vi "BundleMagic.vi"(6 "Mouse Position":cluster{"Left":i32, "Top":i32}, 7 "User VI Ref":refnum<vi>, 8 "Is Multi-select?":bool, 9 "Remaining Items":refnum<vi>[](array[refnum]), 10 "Affected Items":T2, 11 "Menu Refnum":refnum<k9>) -> (3 "Menu Items To Add":T1(array[cluster]))   [LabVIEW 2023]
doc: "This VI is part of a plug-in for modifying the LabVIEW shortcut menus. This is the builder VI which is called when the shortcut menu is built. It tells LabVIEW which shortcut menu items to add to the menu."
uses:
  BundleMagic.ctl
panel:
  # "FIX_NEXT_ISSUE BRANCH"
  # "Rules a popup plug-in must follow:\n* This VI's file name must match the file name of the LLB -- only the file extensions should be different.\n* This VI must have debugging disabled or it will be ignored as a plug-in.\n* For all menu items, \"tag suffix + file name of this VI\" must be less than 240 characters.\n* You can disconnect the \"Affected Items\" from the typedef to make the plug-in load faster. The typedef is only there to assist you in keeping this VI and the execution VI using to the same type.\n* All controls on this panel except \"Affected Items\" are locked to prevent accidental edits. Do not change the types or the names of controls other than the elements inside the \"Affected Items\" cluster.\n* See Context Help for more information on the individual controls."
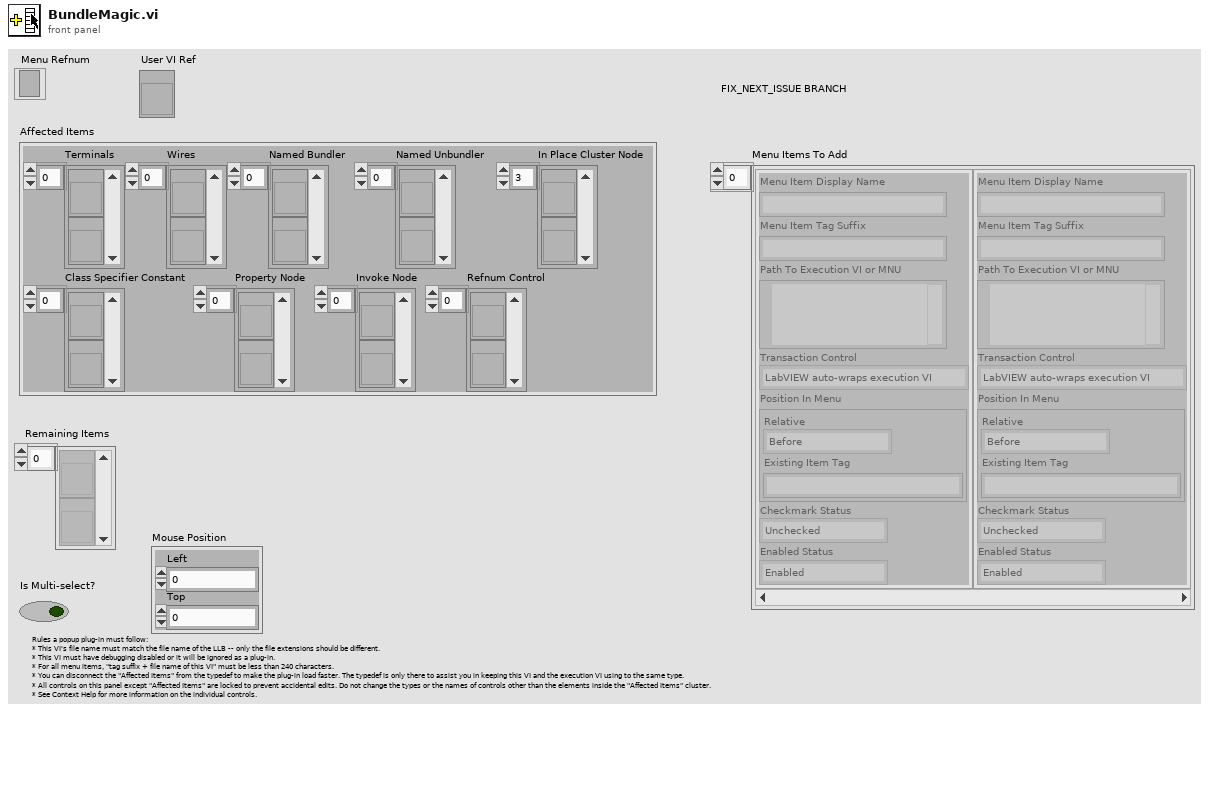
[diagram p1: front panel]
types:
  T1 = cluster{"Menu Item Display Name":string, "Menu Item Tag Suffix":string, "Path To Execution VI or MNU":path, "Transaction Control":enum8{"LabVIEW auto-wraps execution VI", "Execution VI will define if needed"}, "Position In Menu":cluster{"Relative":enum8{"Before", "Instead of", "After", "Into Submenu"}, "Existing Item Tag":string}, "Checkmark Status":enum8{"Unchecked", "Checked"}, "Enabled Status":enum8{"Enabled", "Disabled"}}[]
  T2 = typedef "BundleMagic.ctl" = cluster{"Terminals":refnum<vi>[], "Wires":refnum<vi>[], "Named Bundler":refnum<vi>[], "Named Unbundler":refnum<vi>[], "In Place Cluster Node":refnum<vi>[], "Class Specifier Constant":refnum<vi>[], "Property Node":refnum<vi>[], "Invoke Node":refnum<vi>[], "Refnum Control":refnum<vi>[]}
  T3 = enum16{"[NONE]", "Cluster Wire", "Named Un/Bundler", "In Place", "Cluster Terminal", "Reference Wire", "Reference Terminal", "Property Node", "Class Specifier Constant", "Invoke Node", "Refnum Control"}[]
  T4 = cluster{"Menu Item Display Name":string, "Menu Item Tag Suffix":string, "Path To Execution VI or MNU":path, "Transaction Control":enum8{"LabVIEW auto-wraps execution VI", "Execution VI will define if needed"}, "Position In Menu":cluster{"Relative":enum8{"Before", "Instead of", "After", "Into Submenu"}, "Existing Item Tag":string}, "Checkmark Status":enum8{"Unchecked", "Checked"}, "Enabled Status":enum8{"Enabled", "Disabled"}}
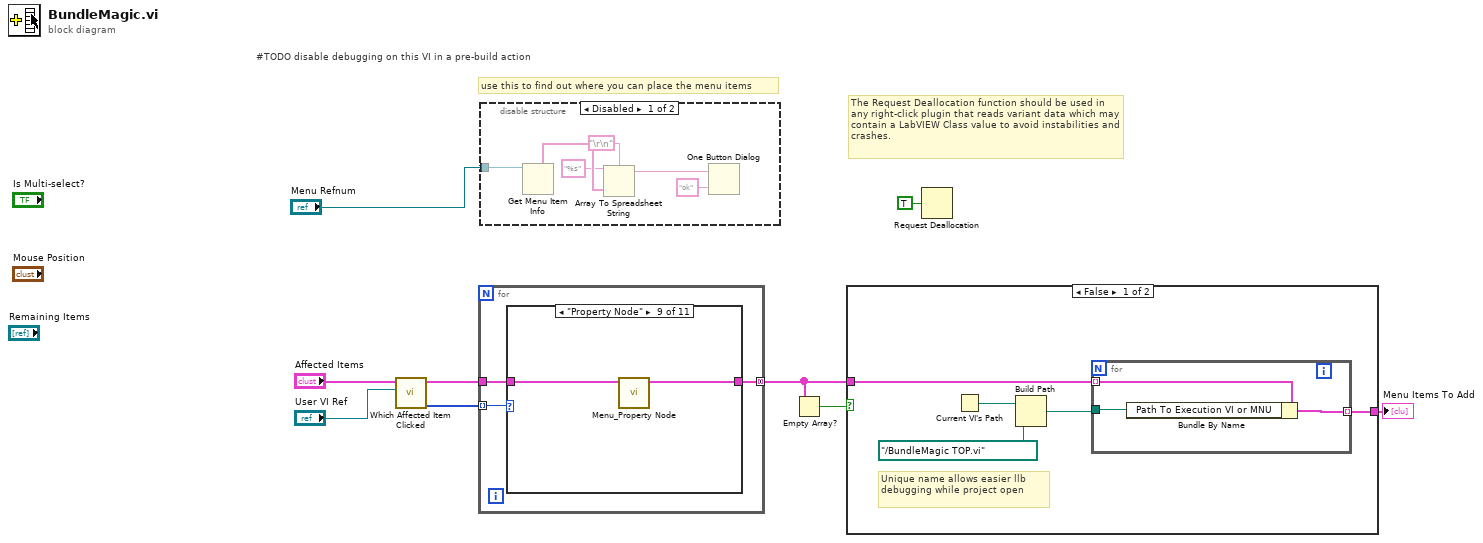
[diagram p0: block diagram]
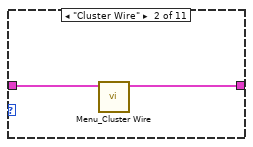
[diagram p3: hidden frame]
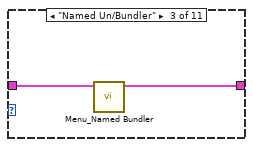
[diagram p4: hidden frame]
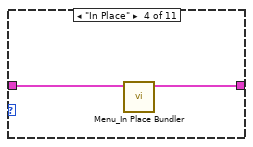
[diagram p5: hidden frame]
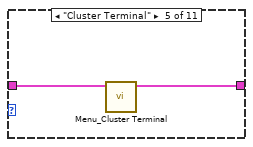
[diagram p6: hidden frame]
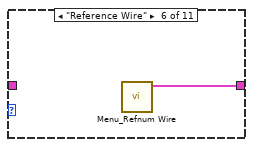
[diagram p7: hidden frame]
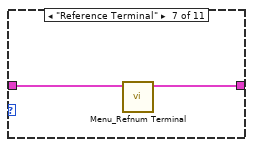
[diagram p8: hidden frame]
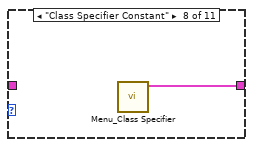
[diagram p9: hidden frame]
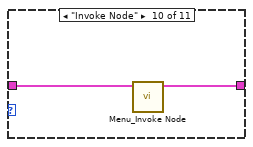
[diagram p10: hidden frame]
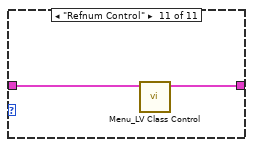
[diagram p11: hidden frame]
diagram:
  # "#TODO disable debugging on this VI in a pre-build action"
  # "use this to find out where you can place the menu items"
  # "The Request Deallocation function should be used in any right-click plugin that reads variant data which may contain a LabVIEW Class value to avoid instabilities and crashes."
  n1 = call "Which Affected Item Clicked.vi"("User VI Ref"="User VI Ref", "Affected Items"="Affected Items") -> ("Compiled Affected Items"=w4:T3, "Affected Items Out"=w5:T2)  [unwired: 7 in, 1 out]
  n2 = for {
    tunnel: [w12] -> w3 mode=concatenating
    tunnel: w5 -> [w11]
    tunnel: w4 -> [w10] mode=indexing
    n3 = case shown="\"Property Node\"" w10 {
      tunnel: [_ w14 w16 w18 w20 w21 w23 w24 w26 w28 w30] -> w12
      tunnel: w11 -> [_ w13 w15 w17 w19 _ w22 _ w25 w27 w29]
      frame "[NONE]" {
      }
      frame "Cluster Wire" {
        n4 = call "Menu_Cluster Wire.vi"("Affected Items"=w13) -> ("Menu Items To Add"=w14:T1)  [unwired: 10 in]
      }
      frame "Named Un/Bundler" {
        n5 = call "Menu_Named Bundler.vi"("Affected Items Out"=w15) -> ("Menu Items To Add"=w16:T1)  [unwired: 10 in]
      }
      frame "In Place" {
        n6 = call "Menu_In Place Bundler.vi"("Affected Items Out"=w17) -> ("Menu Items To Add"=w18:T1)  [unwired: 10 in]
      }
      frame "Cluster Terminal" {
        n7 = call "Menu_Cluster Terminal.vi"("Affected Items"=w19) -> ("Menu Items To Add"=w20:T1)  [unwired: 10 in]
      }
      frame "Reference Wire" {
        n8 = call "Menu_Refnum Wire.vi"() -> ("Menu Items To Add"=w21:T1)  [unwired: 11 in]
      }
      frame "Reference Terminal" {
        n9 = call "Menu_Refnum Terminal.vi"("Affected Items"=w22) -> ("Menu Items To Add"=w23:T1)  [unwired: 10 in]
      }
      frame "Class Specifier Constant" {
        n10 = call "Menu_Class Specifier.vi"() -> ("Menu Items To Add"=w24:T1)  [unwired: 11 in]
      }
      frame "Property Node" {
        n11 = call "Menu_Property Node.vi"("Affected Items Out"=w25) -> ("Menu Items To Add"=w26:T1)  [unwired: 10 in]
      }
      frame "Invoke Node" {
        n12 = call "Menu_Invoke Node.vi"("Affected Items Out"=w27) -> ("Menu Items To Add"=w28:T1)  [unwired: 10 in]
      }
      frame "Refnum Control" {
        n13 = call "Menu_LV Class Control.vi"("Affected Items Out"=w29) -> ("Menu Items To Add"=w30:T1)  [unwired: 10 in]
      }
    }
  }
  n14 = disable-structure shown="Disabled" {
    disable-tunnel: "Menu Refnum" -> [w36 _]
    frame Disabled {
      n15 = Get Menu Item Info(11:w36) -> (5:w34:string[])  [unwired: 2 in, 6 out]
      n16 = Array To Spreadsheet String(delimiter (Tab)="\r\n", array=w34, 3:"%s" ("format string")) -> (spreadsheet string=w31:string)
      n17 = One Button Dialog(message=w31, button name ("OK")="ok" ("message")) -> ()  [unwired: 1 out]
    }
    frame Enabled {
    }
  }
  n18 = Empty Array?(array=w3) -> (empty?=w2:bool)
  n19 = case shown="False" w2 {
    tunnel: [w40 _] -> w8
    tunnel: w3 -> [w37 _]
    frame False {
      # "Unique name allows easier llb debugging while project open"
      n20 = Current VI's Path() -> (path=w41:path)
      n21 = Build Path(base path=w41, name or relative path=path "../BundleMagic TOP.vi" ("execute path")) -> (appended path=w39:path)
      n22 = for {
        tunnel: w39 -> [w44]
        tunnel: [w43] -> w40 mode=indexing
        tunnel: w37 -> [w42] mode=indexing
        n23 = Bundle By Name(cluster=w42, "Path To Execution VI or MNU"=w44) -> (w43:T4)
      }
    }
    frame True {
    }
  }
  "Menu Items To Add" <- w8
  n24 = Request Deallocation(TRUE ("flag")) -> ()
